vi "UI Camera Page.vi"(8 "error in":errorcluster) -> (0 "error out":errorcluster)   [LabVIEW 2019, in "UIs.lvlib"]
uses:
  UIs.lvlib
  LED/SubVI/Image Para.ctl
  MiControl-E/LV Source/ImageSystem/Cradle Zyla_1117/Ctl/seletion.ctl
  <vilib>/Utility/miscctls.llb/LVPointTypeDef.ctl
  Controller/Controller.lvlib
  Camera/Andor/Andor.lvlib
  LED/LED.lvlib
  Motion/Allmotion/Allmotion.lvlib
  Image/Image.lvlib
  Initialize/Initialize.lvlib
panel:
  in  "System Tab":enum32{"Controls", "Acquire Image"}(tab)
  in  "Acquire":bool
  in  "Image Para":T1[](array[typedef])=[{"Marker"=enum."None", "Power(Amp)"=15, "set shutter(s)"=0.05, "Cube"=enum."1"}, {"Marker"=enum."None", "Power(Amp)"=15, "set shutter(s)"=0.05, "Cube"=enum."1"}, {"Marker"=enum."None", "Power(Amp)"=15, "set shutter(s)"=0.05, "Cube"=enum."1"}, {"Marker"=enum."None", "Power(Amp)"=15, "set shutter(s)"=0.05, "Cube"=enum."1"}, {"Marker"=enum."None", "Power(Amp)"=15, "set shutter(s)"=0.05, "Cube"=enum."1"}, {"Marker"=enum."None", "Power(Amp)"=15, "set shutter(s)"=0.05, "Cube"=enum."1"}, {"Marker"=enum."None", "Power(Amp)"=15, "set shutter(s)"=0.05, "Cube"=enum."1"}, {"Marker"=enum."None", "Power(Amp)"=15, "set shutter(s)"=0.05, "Cube"=enum."1"}] {"set shutter(s)" min=0.001 max=3.0 step=0.001; "Power(Amp)" min=15 max=100}
  out "LED Setup":string[][](array[string])=[["Light", "Cube"], ["UV", "2"], ["Red", "3"], ["Green", "4"], ["Blue-Red", "7"], ["Blue", "5"], ["UV-IR", "8"], ["UV-Red", "6"], ["BF", "6"]]
  in  "Back":bool
  # "Light"
  # "Power (%)"
  # "Expo Time (s)"
  # "Cube"
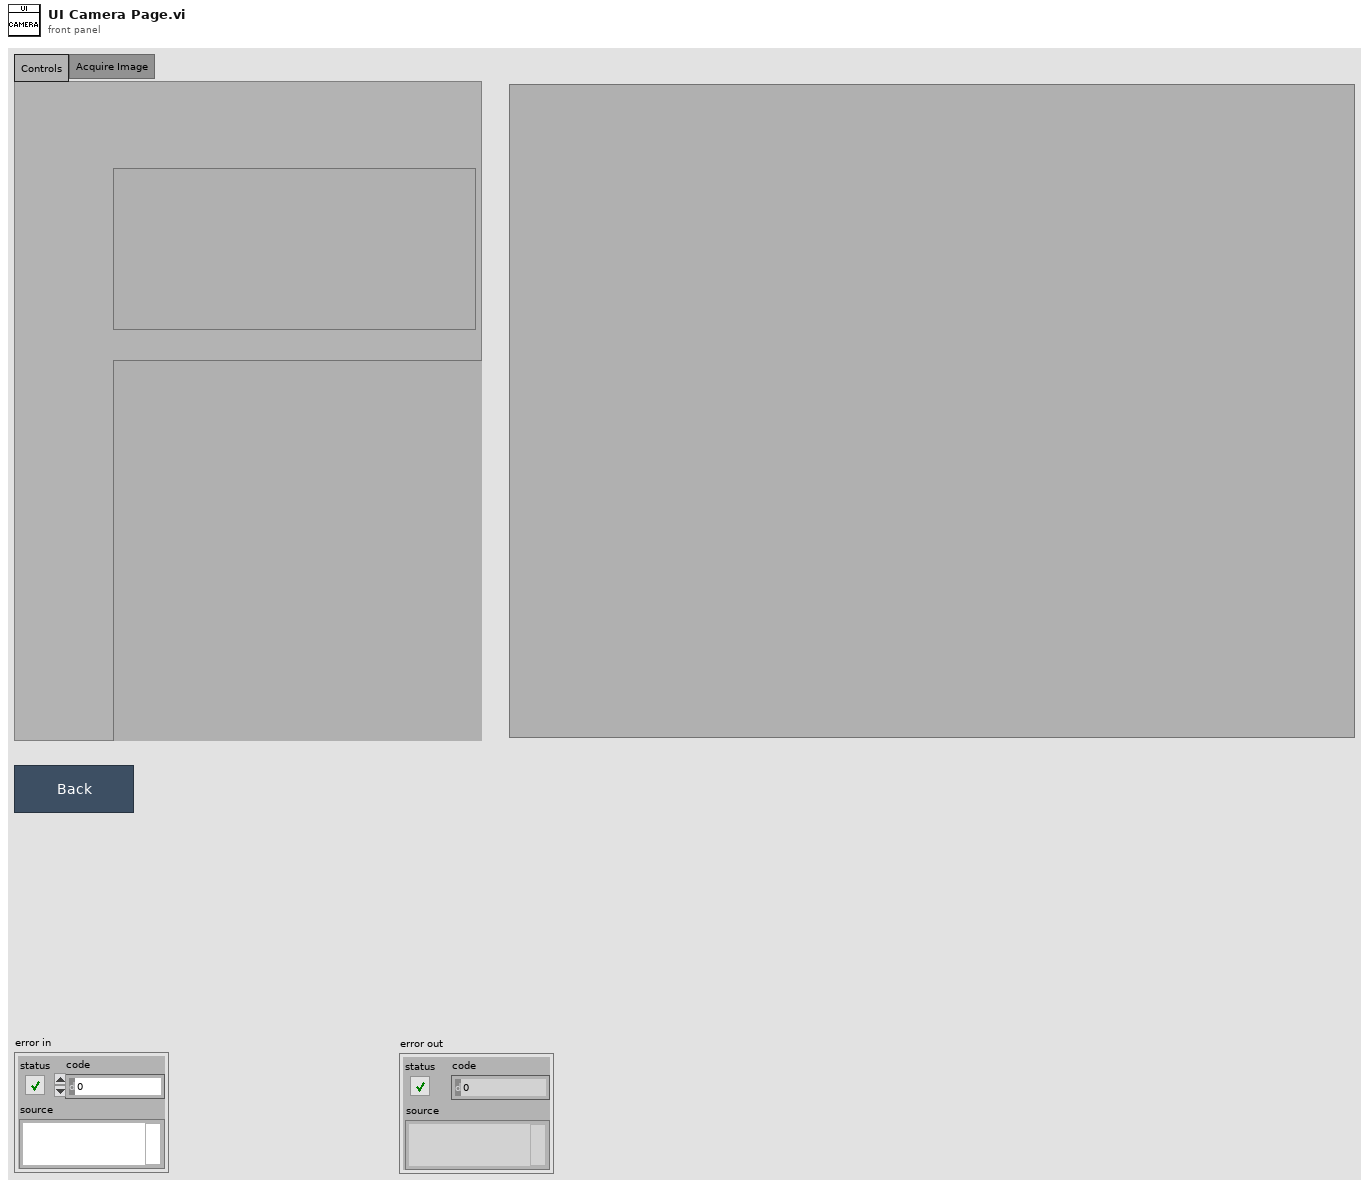
[diagram p1: front panel]
types:
  T1 = typedef "LED.lvlib/Image Para.ctl" = cluster{"Marker":T2, "Power(Amp)":u8, "set shutter(s)":dbl, "Cube":enum16{"1", "2", "3", "4", "5", "6", "7", "8"}}
  T2 = typedef "seletion.ctl" = enum16{"None", "Red", "Green", "Blue", "UV", "Green Laser", "Blue-Red", "UV-Red", "BF", "UV-IR"}
  T3 = typedef "LVPointTypeDef.ctl" = cluster{"Horizontal":i16, "Vertical":i16}
  T4 = typedef "LED.lvlib/SEQ Data.ctl" = cluster{"Initialize Sucess?":bool, "BL2 Regulator":dbl, "BL1 Regulator":dbl, "Blood Sensor 1":dbl, "Blood Sensor 2":dbl, "Air Pressure Sensor":dbl, "Force Snesor 1":u32, "Force Snesor 2":u32, "VI Refnum":refnum<vi>}
  T5 = typedef "Andor.lvlib/SEQ Data.ctl" = cluster{"Initialize Sucess?":bool, "Image Ref":T6, "VI Refnum":refnum<vi>}
  T6 = typedef "IMAQ Image.ctl" = refnum<image>
  T7 = typedef "Allmotion.lvlib/SEQ Data.ctl" = cluster{"Position":i32[], "Arrived?":bool, "VISA name":refnum<visa-resource-name>, "Initialize Done?":bool, "State":string, "VI Refnum":refnum<vi>, "Dichroic Position":string[]}
  T8 = typedef "Initialize.lvlib/SEQ Data.ctl" = cluster{"Folder Path":path}
  T9 = typedef "Image.lvlib/SEQ Data.ctl" = cluster{"Acquire Done?":bool, "Focus Done?":bool, "Align Done?":bool, "No Position Match?":bool, "Best Wheel Position":string, "Match Done?":bool, "Match Score":dbl, "Focus Score":dbl, "Match Position":cluster{"x":sgl, "y":sgl}, "Flower Position":i32[]}
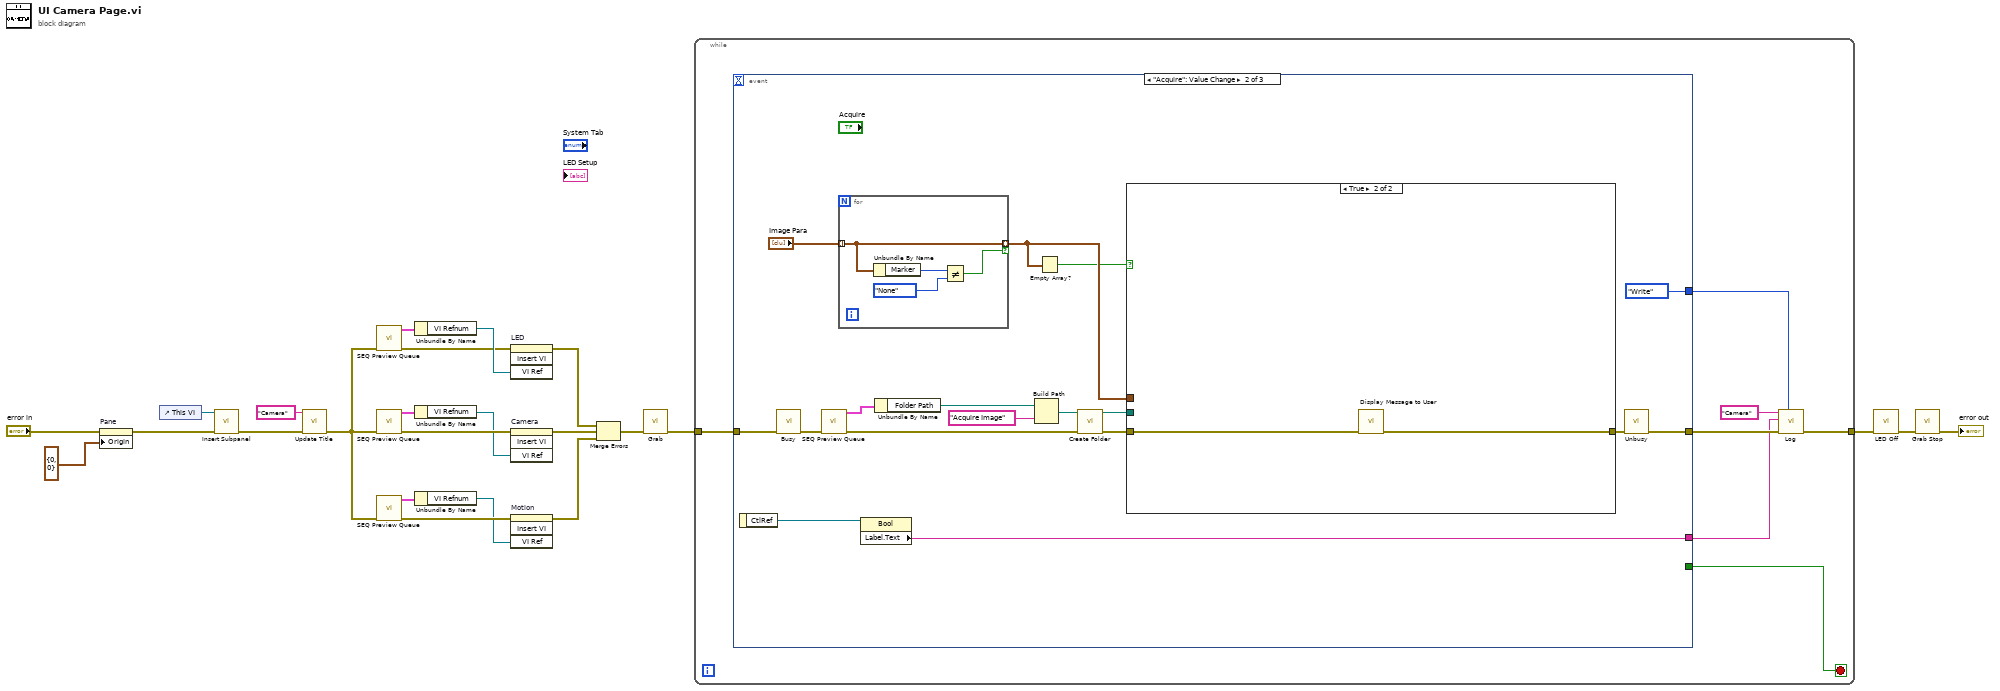
[diagram p0: block diagram]
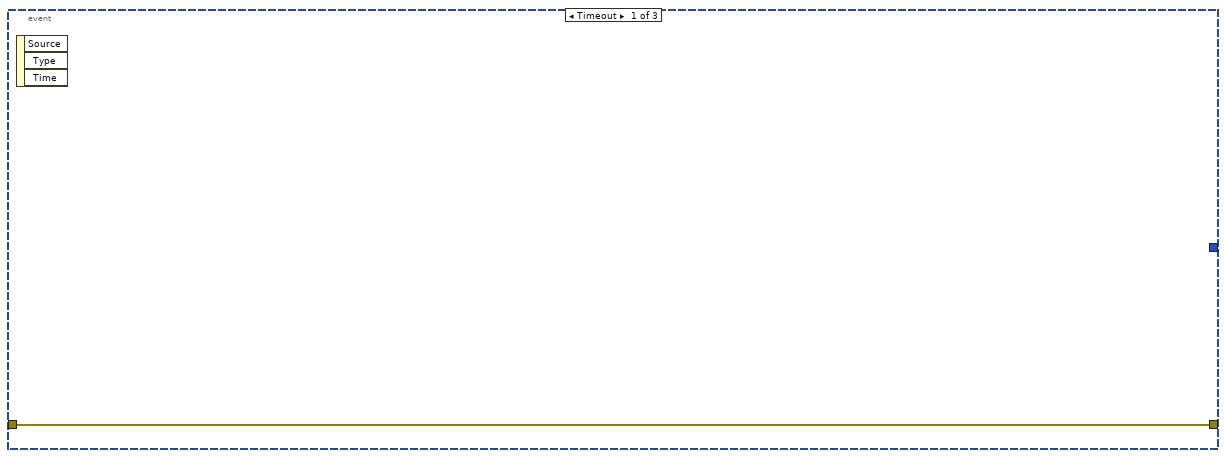
[diagram p2: hidden frame]
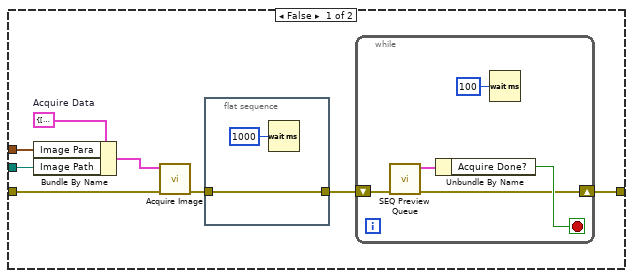
[diagram p3: hidden frame]
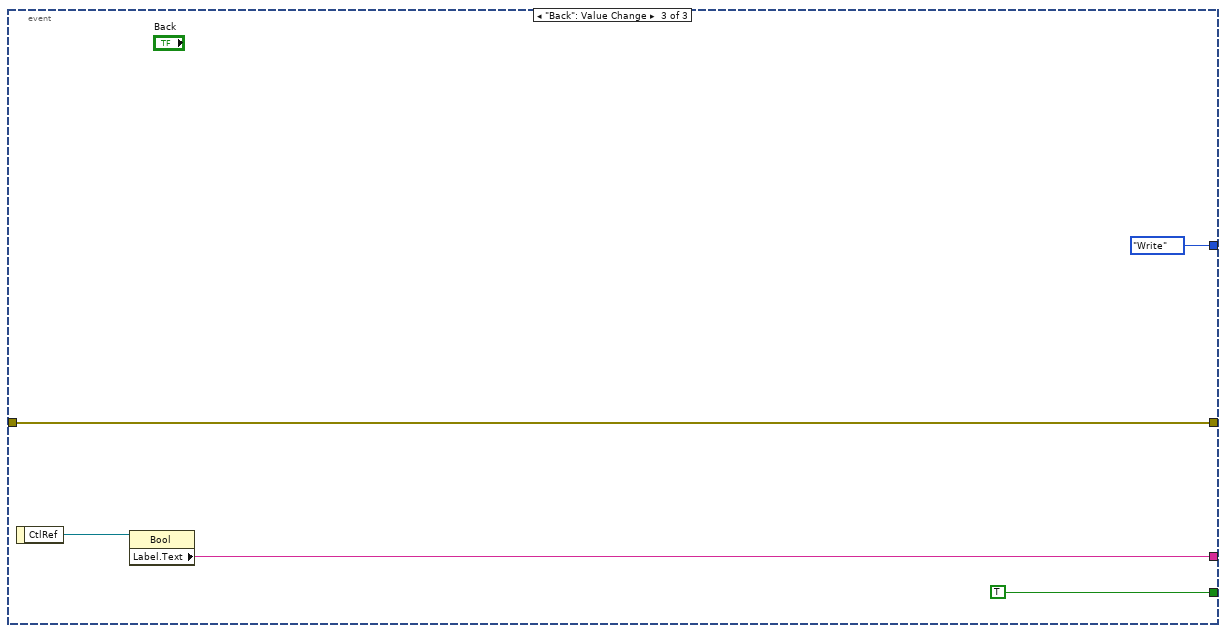
[diagram p4: hidden frame]
diagram:
  n1 = property on="Pane" class="Pane"(error in="error in", "Origin"=T3 {"Horizontal"=0, "Vertical"=0}) -> (error out=w10:errorcluster)  [unwired: 1 in, 1 out]
  n2 = control-ref of="This VI"() -> (w24:refnum<vi>)
  n3 = call "Insert Subpanel.vi"("Error In"=w10, "VI Refnum"=w24) -> ("Error Out"=w3:errorcluster)  [unwired: 9 in]
  n4 = call "Update Title.vi"("Error In"=w3, "Title"="Camera") -> ("Error Out"=w2:errorcluster)  [unwired: 9 in]
  n5 = call "SEQ Preview Queue.vi"("error in"=w2) -> ("error out"=w15:errorcluster, "SEQ Data"=w19:T4)  [unwired: 9 in]
  n6 = call "SEQ Preview Queue.vi"("error in"=w2) -> ("error out"=w23:errorcluster, "SEQ Data"=w22:T5)  [unwired: 9 in]
  n7 = call "SEQ Preview Queue.vi"("error in"=w2) -> ("error out"=w18:errorcluster, "SEQ Data"=w20:T7)  [unwired: 9 in]
  n8 = Unbundle By Name(w19) -> ("VI Refnum"=w16:refnum<vi>)
  n9 = Unbundle By Name(w22) -> ("VI Refnum"=w21:refnum<vi>)
  n10 = Unbundle By Name(w20) -> ("VI Refnum"=w17:refnum<vi>)
  n11 = invoke on="LED" class="SubPnl" method="Insert VI"(error in=w15, "VI Ref"=w16) -> (error out=w14:errorcluster)  [unwired: 2 in, 3 out]
  n12 = invoke on="Camera" class="SubPnl" method="Insert VI"(error in=w23, "VI Ref"=w21) -> (error out=w13:errorcluster)  [unwired: 2 in, 3 out]
  n13 = invoke on="Motion" class="SubPnl" method="Insert VI"(error in=w18, "VI Ref"=w17) -> (error out=w12:errorcluster)  [unwired: 2 in, 3 out]
  n14 = Merge Errors(w14, w13, w12) -> (w8:errorcluster)
  n15 = call "Grab.vi"("Error In"=w8) -> ("Error Out"=w7:errorcluster)  [unwired: 10 in]
  n16 = while {
    tunnel: w7 -> [w31]
    tunnel: [w28] -> w5
    stop <- w30 stop-if-true
    n17 = event shown="[1] \"Acquire\": Value Change" {
      selector: _ -> [_ _ _]
      dyn-events: _ -> [_ _ _]
      timeout: _ -> [_ _ _]
      tunnel: w31 -> [w32 w42 w75]
      tunnel: [w32 w39 w75] -> w29
      tunnel: [_ _ TRUE] -> w30
      tunnel: [_ enum16{"None", "Write"}."Write" ("Action") enum16{"None", "Write"}."Write" ("Action")] -> w26
      tunnel: [_ w33 w71] -> w25
      event Timeout {
        n18 = event-data() -> ()  [unwired: 1 in, 3 out]
      }
      event "Acquire": Value Change {
        n19 = event-data() -> ("CtlRef"=w34:refnum<vi>)  [unwired: 1 in]
        n20 = call "Busy.vi"("Error In"=w42) -> ("Error Out"=w41:errorcluster)  [unwired: 10 in]
        n21 = call "SEQ Preview Queue.vi"("error in"=w41) -> ("error out"=w45:errorcluster, "SEQ Data"=w44:T8)  [unwired: 9 in]
        n22 = for {
          tunnel: "Image Para" -> [w68] mode=indexing
          tunnel: [w68] -> w37 mode=indexing if=w67
          n23 = Unbundle By Name(w68) -> ("Marker"=w70:T2)
          n24 = Not Equal?(x=w70, y=seletion."None" ("Marker")) -> (x != y?=w67:bool)
        }
        n25 = property class="Bool"(reference=w34) -> ("Label.Text"=w33:string)  [unwired: 1 in, 2 out]
        n26 = Unbundle By Name(w44) -> ("Folder Path"=w43:path)
        n27 = Build Path(base path=w43, name or relative path="Acquire Image") -> (appended path=w46:path)
        n28 = Empty Array?(array=w37) -> (empty?=w36:bool)
        n29 = call "Create Folder.vi"("error in"=w45, "Path in"=w46) -> ("error out"=w48:errorcluster, "Path out"=w47:path)  [unwired: 8 in]
        n30 = case shown="True" w36 {
          tunnel: w48 -> [w53 w66]
          tunnel: w47 -> [w52 _]
          tunnel: [w51 w65] -> w40
          tunnel: w37 -> [w50 _]
          frame False {
            w54 = cluster{"Image Para":T1[], "Image Path":path} {"Image Para"=[], "Image Path"=path ""}  # Acquire Data
            n31 = Bundle By Name(cluster=w54, "Image Para"=w50, "Image Path"=w52) -> (w55:cluster{"Image Para":T1[], "Image Path":path})
            n32 = call "Acquire Image.vi"("Error In"=w53, "Acquire Data"=w55) -> ("Error Out"=w56:errorcluster)  [unwired: 9 in]
            n33 = flat-sequence {
              tunnel: w56 -> [w63]
              tunnel: [w63] -> w57
              frame #0 {
                n34 = Wait (ms)(milliseconds to wait=u32 1000) -> ()  [unwired: 1 out]
              }
            }
            n35 = while {
              shift-right: [w58] -> w51
              shift-left: w57 -> [w62]
              stop <- w59 stop-if-true
              n36 = call "SEQ Preview Queue.vi"("error in"=w62) -> ("error out"=w58:errorcluster, "SEQ Data"=w60:T9)  [unwired: 9 in]
              n37 = Unbundle By Name(w60) -> ("Acquire Done?"=w59:bool)
              n38 = Wait (ms)(milliseconds to wait=u32 100) -> ()  [unwired: 1 out]
            }
          }
          frame True {
            n39 = call "Display Message to User"("error in (no error)"=w66) -> ("error out"=w65:errorcluster)  [unwired: 9 in, 1 out]
          }
        }
        n40 = call "Unbusy.vi"("Error In"=w40) -> ("Error Out"=w39:errorcluster)  [unwired: 10 in]
      }
      event "Back": Value Change {
        n41 = event-data() -> ("CtlRef"=w72:refnum<vi>)  [unwired: 1 in]
        n42 = property class="Bool"(reference=w72) -> ("Label.Text"=w71:string)  [unwired: 1 in, 2 out]
      }
    }
    n43 = call "Log.vi"("Action"=w26, "error in"=w29, "State"=w25, "Page Name"="Camera") -> ("error out"=w28:errorcluster)  [unwired: 7 in]
  }
  n44 = call "LED Off.vi"("Error In"=w5) -> ("Error Out"=w4:errorcluster)  [unwired: 10 in]
  n45 = call "Grab Stop.vi"("Error In"=w4) -> ("Error Out"=→"error out":errorcluster)  [unwired: 10 in]
